vi "ReadAllPositions.vi"(8 "error in (no error)":errorcluster, 11 "VXMx2 in":refnum<class "VXMx2.lvclass">) -> (0 "error out":errorcluster, 1 "Z, eng units":dbl, 2 "Y, eng units":dbl, 3 "VXMx2 out":refnum<class "VXMx2.lvclass">, 4 "T, eng units":dbl, 5 "X, eng units":dbl, 6 "sub-syst.VXM (1-4)":i32, 7 "All Positions, eng units":dbl[](array[numeric]))   [LabVIEW 2019, in "VXMx2.lvclass"]
doc: "read positions from VXM.\nThis VI should be called when there's no motion becauset the VXM2 can't read Z and T when in motion."
uses:
  VXMx2.lvclass
  VXMx2.lvclass/VXMx2.ctl
  <instrlib>/Velmex VXM/Velmex VXM.lvlib
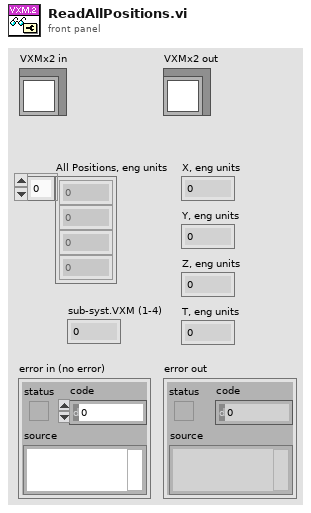
[diagram p1: front panel]
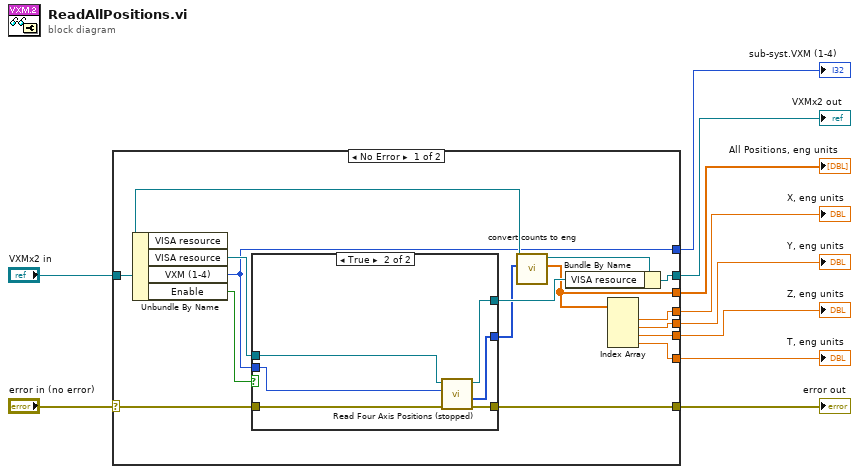
[diagram p0: block diagram]
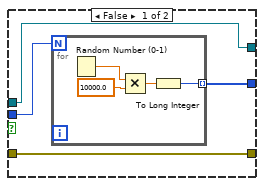
[diagram p2: hidden frame]
diagram:
  n1 = case shown="No Error" "error in (no error)" {
    selector: "error in (no error)" -> [w19 w41]
    tunnel: [w18 w41] -> w9
    tunnel: [w25 w40] -> w7
    tunnel: "VXMx2 in" -> [w15 w40]
    tunnel: [w23 _] -> w6
    tunnel: [w22 _] -> w2
    tunnel: [w21 _] -> w5
    tunnel: [w20 _] -> w4
    tunnel: [w13 _] -> w3
    tunnel: [w11 _] -> w1
    frame No Error {
      n2 = Unbundle By Name(w15) -> ("VISA resource"=w12:refnum<visa-resource-name>, "VXM (1-4)"=w11:i32, "Enable"=w17:bool)  [unwired: 1 out]
      n3 = case shown="True" w17 {
        tunnel: w11 -> [w26 w35]
        tunnel: [w29 w39] -> w16
        tunnel: [w27 w38] -> w24
        tunnel: w19 -> [w28 w37]
        tunnel: [w28 w36] -> w18
        tunnel: w12 -> [w27 w34]
        frame False {
          n4 = for {
            N: w26 -> [_]
            tunnel: [w30] -> w29 mode=indexing
            n5 = Random Number (0-1)() -> (number: 0 to 1=w33:dbl)
            n6 = Multiply(x=w33, y=10000.0) -> (x*y=w31:dbl)
            n7 = To Long Integer(number=w31) -> (32bit integer=w30:i32)
          }
        }
        frame True {
          n8 = call <instrlib>:"Read Four Axis Positions (stopped).vi"("error in (no error)"=w37, "VXM Model (1-4)"=w35, "VISA resource name"=w34) -> ("error out"=w36:errorcluster, "Positions, counts"=w39:i32[], "VISA resource out"=w38:refnum<visa-resource-name>)  [unwired: 6 in]
        }
      }
      n9 = call "convert counts to eng.vi"("All Positions, counts"=w16, "VXMx2 in"=w15) -> ("All Positions, eng units"=w13:dbl[], "VXMx2 out"=w14:refnum<class "VXMx2.lvclass">)  [unwired: 6 in, 2 out]
      n10 = Bundle By Name(cluster=w14, "VISA resource"=w24) -> (w25:refnum<class "VXMx2.lvclass">)
      n11 = Index Array(array=w13) -> (element #1=w23:dbl, element #2=w22:dbl, element #3=w21:dbl, element #4=w20:dbl)  [unwired: 4 in]
    }
    frame Error {
    }
  }
  "error out" <- w9
  "VXMx2 out" <- w7
  "Y, eng units" <- w2
  "Z, eng units" <- w5
  "T, eng units" <- w4
  "X, eng units" <- w6
  "All Positions, eng units" <- w3
  "sub-syst.VXM (1-4)" <- w1
